vi "Type.Determine.vi"(8 "error in (no error)":errorcluster, 11 "Node Ptr":u64) -> (0 "error out":errorcluster, 1 "Found?":bool, 2 "Type":T2, 3 "Item Ref out":T1 format="%.0x")   [LabVIEW 2019, in "Diagnostics Addon System Explorer.lvlib"]
uses:
  Shared/Types/Type.ctl
  <vilib>/NI VeriStand/Custom Device API/Custom Device Item Ref.ctl
  Shared/SubVIs/Constants.vi
  Diagnostics Addon System Explorer.lvlib
  <vilib>/NI VeriStand/Custom Device API/Custom Device API.lvlib
  Shared/Diagnostics Addon Shared.lvlib
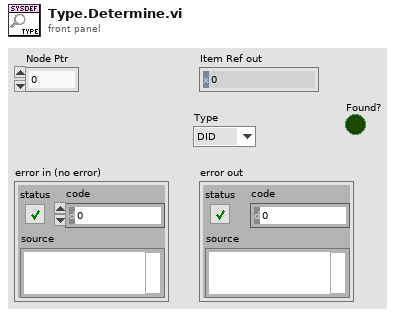
[diagram p1: front panel]
types:
  T1 = typedef "Custom Device API.lvlib/Custom Device Item Ref.ctl" = u64
  T2 = typedef "Diagnostics Addon Shared.lvlib/Type.ctl" = enum16{"DID", "CDID", "PID", "CPID", "Read Memory", "Write Memory", "IO Control", "Routine Start", "Routine Request", "Routine Stop", "User Defined", "DTC Control", "Clear DTCs", "Read DTCs", "Start DTCs", "DTC Change Count", "Tester Present", "Unlock ECU", "Reset ECU", "Diagnostic Session Control", "Normal Communication Control", "Configure and Start DPIDs", "Stop DPIDs"}
  T3 = typedef "Custom Device API.lvlib/Custom Device Item Info.ctl" = cluster{"Name":string, "Is Channel":bool, "GUID":string, "Is Waveform":bool}
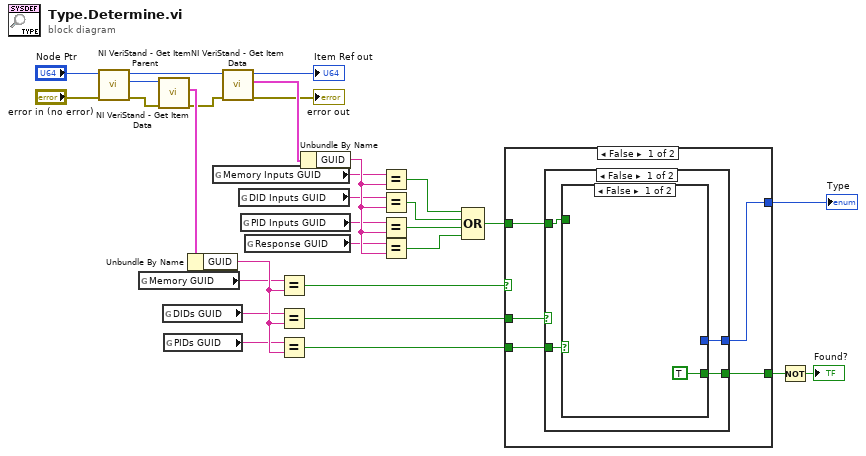
[diagram p0: block diagram]
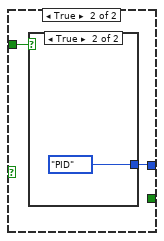
[diagram p2: hidden frame]
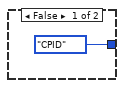
[diagram p3: hidden frame]
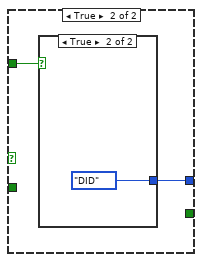
[diagram p4: hidden frame]
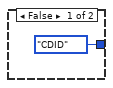
[diagram p5: hidden frame]
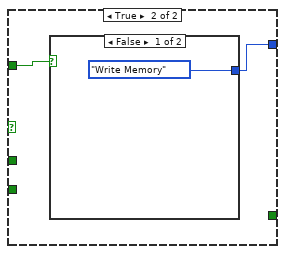
[diagram p6: hidden frame]
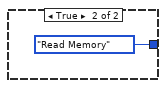
[diagram p7: hidden frame]
diagram:
  n1 = call <vilib>:"NI VeriStand - Get Item Parent.vi"("error in (no error)"="error in (no error)", "Item Ref in"="Node Ptr") -> ("error out"=w16:errorcluster, "Parent Ref"=w15:T1, "Item Ref out"=w14:T1)  [unwired: 6 in, 1 out]
  n2 = global read "Constants.vi" "Memory GUID"() -> (w19:string)
  n3 = call <vilib>:"NI VeriStand - Get Item Data.vi"("error in (no error)"=w16, "Item Ref in"=w15) -> ("error out"=w17:errorcluster, "Item Info"=w18:T3)  [unwired: 6 in, 2 out]
  n4 = global read "Constants.vi" "DIDs GUID"() -> (w20:string)
  n5 = global read "Constants.vi" "PIDs GUID"() -> (w21:string)
  n6 = Unbundle By Name(w18) -> ("GUID"=w22:string)
  n7 = global read "Constants.vi" "Memory Inputs GUID"() -> (w8:string)
  n8 = call <vilib>:"NI VeriStand - Get Item Data.vi"("error in (no error)"=w17, "Item Ref in"=w14) -> ("error out"=→"error out":errorcluster, "Item Info"=w5:T3, "Item Ref out"=→"Item Ref out":T1)  [unwired: 6 in, 1 out]
  n9 = global read "Constants.vi" "DID Inputs GUID"() -> (w7:string)
  n10 = global read "Constants.vi" "PID Inputs GUID"() -> (w6:string)
  n11 = global read "Constants.vi" "Response GUID"() -> (w28:string)
  n12 = Equal?(x=w19, y=w22) -> (x = y?=w25:bool)
  n13 = Equal?(x=w20, y=w22) -> (x = y?=w24:bool)
  n14 = Equal?(x=w21, y=w22) -> (x = y?=w23:bool)
  n15 = Unbundle By Name(w5) -> ("GUID"=w29:string)
  n16 = Equal?(x=w8, y=w29) -> (x = y?=w11:bool)
  n17 = Equal?(x=w7, y=w29) -> (x = y?=w10:bool)
  n18 = Equal?(x=w6, y=w29) -> (x = y?=w9:bool)
  n19 = Equal?(x=w28, y=w29) -> (x = y?=w30:bool)
  n20 = Compound Arithmetic op=OR(w11, w10, w9, w30) -> (w26:bool)
  n21 = case shown="False" w25 {
    tunnel: w23 -> [w35 _]
    tunnel: w24 -> [w34 _]
    tunnel: [w33 w50] -> w27
    tunnel: w26 -> [w32 w49]
    tunnel: [w31 _] -> w2
    frame False {
      n22 = case shown="False" w34 {
        tunnel: w35 -> [w39 _]
        tunnel: [w38 w46] -> w33
        tunnel: w32 -> [w37 w45]
        tunnel: [w36 _] -> w31
        frame False {
          n23 = case shown="False" w39 {
            tunnel: [_ w42] -> w38
            tunnel: w37 -> [_ w41]
            tunnel: [TRUE _] -> w36
            frame False {
            }
            frame True {
              n24 = case shown="True" w41 {
                tunnel: [Type."CPID" ("Type") Type."PID" ("Type")] -> w42
                frame False {
                }
                frame True {
                }
              }
            }
          }
        }
        frame True {
          n25 = case shown="True" w45 {
            tunnel: [Type."CDID" ("Type") Type."DID" ("Type")] -> w46
            frame False {
            }
            frame True {
            }
          }
        }
      }
    }
    frame True {
      n26 = case shown="False" w49 {
        tunnel: [Type."Write Memory" ("Type") Type."Read Memory" ("Type")] -> w50
        frame False {
        }
        frame True {
        }
      }
    }
  }
  "Type" <- w27
  n27 = Not(x=w2) -> (.not. x?=→"Found?":bool)
